vi "Create Library.vi"(8 "error in (no error)":errorcluster, 9 "Music Element Library":refnum<class "MusicElement.lvclass">[](array[class]), 10 "Name":string, 11 "MusicElementLibrary in":refnum<class "MusicElementLibrary.lvclass">) -> (0 "error out":errorcluster, 3 "MusicElementLibrary out":refnum<class "MusicElementLibrary.lvclass">)   [LabVIEW 2015, in "MusicElementLibrary.lvclass"]
uses:
  MusicElementLibrary.lvclass
  MusicElement.lvclass
  MusicElementLibrary.lvclass/MusicElementLibrary.ctl
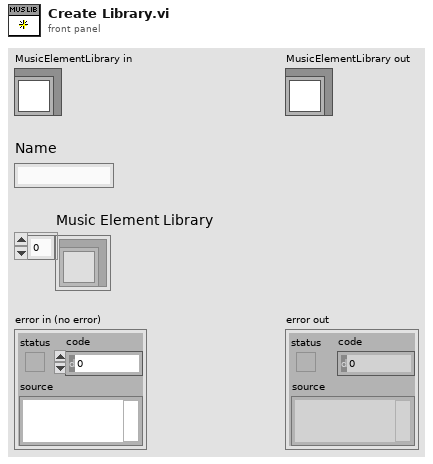
[diagram p1: front panel]
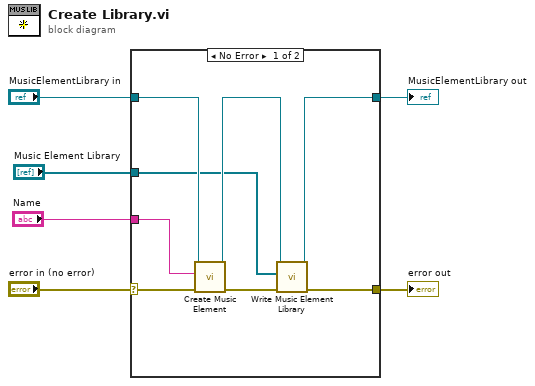
[diagram p0: block diagram]
diagram:
  n1 = case shown="No Error" "error in (no error)" {
    selector: "error in (no error)" -> [w14 w16]
    tunnel: [w7 w16] -> w5
    tunnel: [w9 w15] -> w3
    tunnel: "MusicElementLibrary in" -> [w12 w15]
    tunnel: "Name" -> [w13 _]
    tunnel: "Music Element Library" -> [w8 _]
    frame No Error {
      n2 = call "Create Music Element.vi"("error in (no error)"=w14, "Name"=w13, "MusicElement in"=w12) -> ("error out"=w11:errorcluster, "MusicElement out"=w10:refnum<class "MusicElementLibrary.lvclass">)  [unwired: 7 in]
      n3 = call "Write Music Element Library.vi"("error in (no error)"=w11, "Music Element Library"=w8, "MusicElementLibrary in"=w10) -> ("error out"=w7:errorcluster, "MusicElementLibrary out"=w9:refnum<class "MusicElementLibrary.lvclass">)  [unwired: 7 in]
    }
    frame Error {
    }
  }
  "error out" <- w5
  "MusicElementLibrary out" <- w3
